vi "LOGIC_dcs.vi"(0 "image ptrs (reset - expo - subs)":u64[](array[numeric]), 1 "TotalPixels":u32, 2 "inverse":bool, 6 "write to disk":bool, 7 "Database RefNum out 2":T1, 8 "Log File":path, 9 "name":string, 11 "error in (no error)":errorcluster, 12 "reset and expo bpp":u8=16) -> (4 "image ptrs (reset - expo - subs) out":u64[](array[numeric]), 5 "bpp":i16, 10 "unsc buffer":u64, 15 "error out":errorcluster)   [LabVIEW 2016]
uses:
  DBSHAND/private/vis/DatabaseHand_RefNum.ctl
  Common/public/vis/CMN_FVAR_action.ctl
  DBSHAND/private/vis/DatabaseHand_Element_Get(bool).vi
  DBSHAND/private/vis/DatabaseHand_Element_Set(single).vi
  public/c/lib/libLogic.so
panel:
  out "output ptr (subs image)":u64
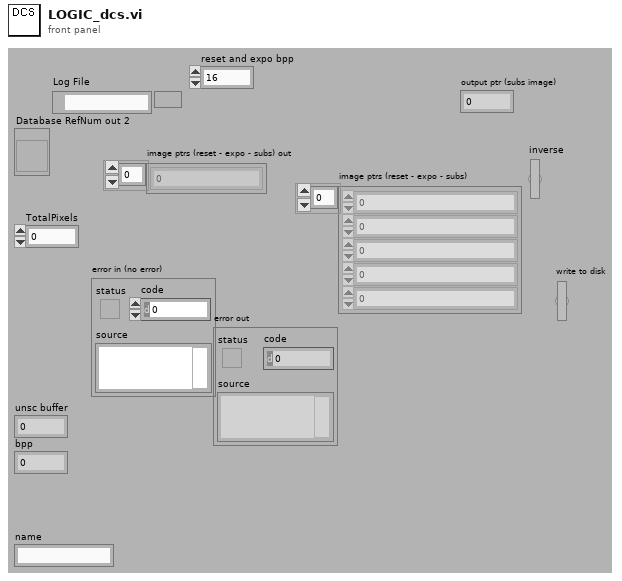
[diagram p1: front panel]
types:
  T1 = typedef "DatabaseHand_RefNum.ctl" = refnum<vi>
  T2 = typedef "CMN_FVAR_action.ctl" = enum16{"read", "write"}
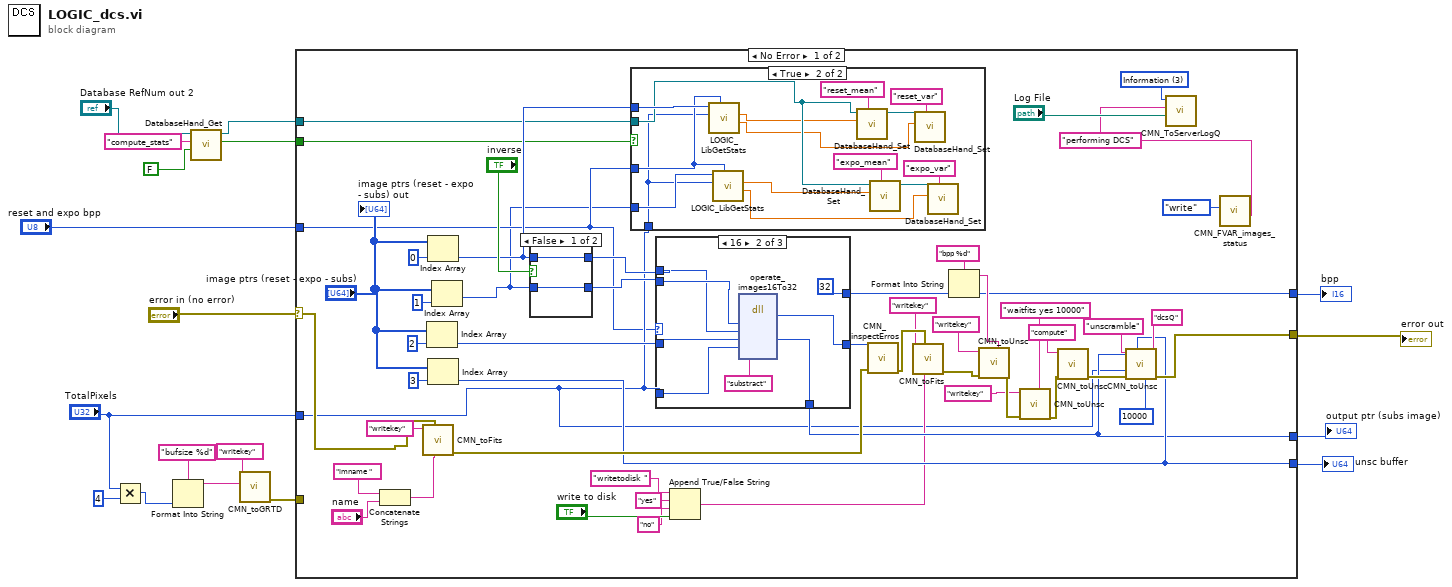
[diagram p0: block diagram]
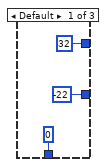
[diagram p4: hidden frame]
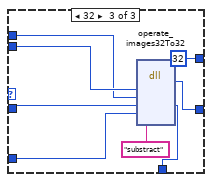
[diagram p5: hidden frame]
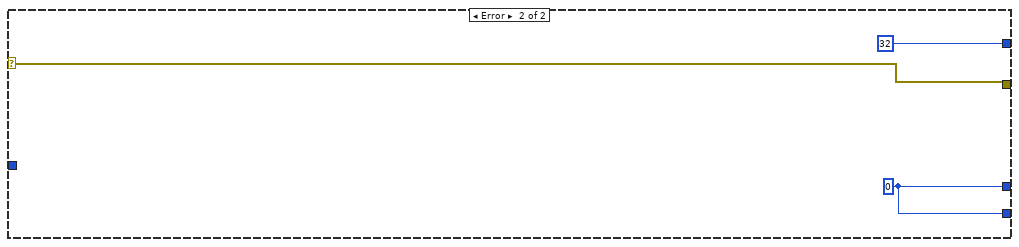
[diagram p6: hidden frame]
diagram:
  n1 = Multiply(x="TotalPixels", y=u32 4) -> (x*y=w12:u32)
  n2 = Format Into String(format string="bufsize %d", w12) -> (resulting string=w11:string)  [unwired: 2 in, 1 out]
  n3 = call-poly "DatabaseHand_Get.vi"("default value"=FALSE, "name"="compute_stats", "Database RefNum in"="Database RefNum out 2") -> ("value"=w2:bool, "Database RefNum out"=w1:T1)  [unwired: 2 in, 5 out]
  n4 = call "CMN_toGRTD.vi"("argument"=w11, "Command"="writekey") -> ("error out"=w10:errorcluster)  [unwired: 6 in, 3 out]
  n5 = case shown="No Error" "error in (no error)" {
    selector: "error in (no error)" -> [w48 w109]
    tunnel: [w65 w109] -> w7
    tunnel: "TotalPixels" -> [w23 _]
    tunnel: [w41 w108] -> w18
    tunnel: [w42 w108] -> w17
    tunnel: w10 -> [_ _]
    tunnel: [w30 32] -> w9
    tunnel: "reset and expo bpp" -> [w22 _]
    tunnel: w2 -> [w21 _]
    tunnel: w1 -> [w20 _]
    frame No Error {
      w52 = u16 3 items=["command", "imediateReply", "Callback Reply", "Information"] ("type")
      w26 = "performing DCS" ("image status")
      n6 = Concatenate Strings("imname " ("key"), "name") -> (w44:string)
      n7 = call "CMN_toFits.vi"("key"=w44, "error in (no error)"=w48, "command"="writekey") -> ("error out"=w47:errorcluster)  [unwired: 5 in, 3 out]
      n8 = Index Array(array="image ptrs (reset - expo - subs)", index=2 ("Index")) -> (element=w51:u64)
      n9 = Index Array(array="image ptrs (reset - expo - subs)", index=0 ("Index")) -> (element=w24:u64)
      n10 = Index Array(array="image ptrs (reset - expo - subs)", index=3 ("Index")) -> (element=w42:u64)
      n11 = Index Array(array="image ptrs (reset - expo - subs)", index=1 ("Index")) -> (element=w19:u64)
      n12 = case shown="False" "inverse" {
        tunnel: w24 -> [w85 w87]
        tunnel: [w85 w86] -> w28
        tunnel: w19 -> [w84 w86]
        tunnel: [w84 w87] -> w27
        frame False {
        }
        frame True {
        }
      }
      n13 = case shown="True" w21 {
        tunnel: w24 -> [_ w83]
        tunnel: w23 -> [_ w73]
        tunnel: w22 -> [_ w74]
        tunnel: w20 -> [_ w76]
        tunnel: w19 -> [_ w75]
        frame False {
        }
        frame True {
          n14 = call "LOGIC_LibGetStats.vi"("bpp"=w74, "num_elems"=w73, "imageptr"=w83) -> ("var"=w69:sgl, "mean"=w70:sgl)  [unwired: 7 out]
          n15 = call "LOGIC_LibGetStats.vi"("bpp"=w74, "num_elems"=w73, "imageptr"=w75) -> ("var"=w71:sgl, "mean"=w72:sgl)  [unwired: 7 out]
          n16 = call-poly "DatabaseHand_Set.vi"("name"="reset_mean", "value"=w70, "Database RefNum in"=w76) -> ("Database RefNum out"=w82:T1)  [unwired: 5 in, 3 out]
          n17 = call-poly "DatabaseHand_Set.vi"("name"="expo_mean", "value"=w72, "Database RefNum in"=w76) -> ("Database RefNum out"=w79:T1)  [unwired: 5 in, 3 out]
          n18 = call-poly "DatabaseHand_Set.vi"("name"="reset_var", "value"=w69, "Database RefNum in"=w82) -> ()  [unwired: 5 in, 4 out]
          n19 = call-poly "DatabaseHand_Set.vi"("name"="expo_var", "value"=w71, "Database RefNum in"=w79) -> ()  [unwired: 5 in, 4 out]
        }
      }
      n20 = case shown="16" w22 {
        tunnel: w23 -> [_ w98 w106]
        tunnel: w51 -> [_ w92 w100]
        tunnel: w28 -> [_ w93 w101]
        tunnel: w27 -> [_ w94 w102]
        tunnel: [-22 w96 w104] -> w63
        tunnel: [32 32 32] -> w30
        tunnel: [u64 0 ("imageptr3") w91 w99] -> w41
        frame Default {
        }
        frame 16 {
          n21 = dll-call lib="home/simager/panview/PAN/Modules/Logical/public/c/lib/libLogic.so" fn="operate_images16To32"("image1ptr"=w94, "image2ptr"=w93, "imageptr3"=w92, "num_elems"=w98, "operation"="substract") -> ("return type"=w96:i32, "imageptr3"=w91:u64)  [unwired: 6 in, 3 out]
        }
        frame 32 {
          n22 = dll-call lib="home/simager/panview/PAN/Modules/Logical/public/c/lib/libLogic.so" fn="operate_images32To32"("image1ptr"=w102, "image2ptr"=w101, "imageptr3"=w100, "num_elems"=w106, "operation"="substract") -> ("return type"=w104:i32, "imageptr3"=w99:u64)  [unwired: 6 in, 3 out]
        }
      }
      n23 = Append True/False String(1:"write to disk", 2:"no" ("false string"), 3:"yes" ("true string"), 4:"writetodisk " ("string (\"\")")) -> (0:w31:string)
      n24 = call "CMN_inspectErros.vi"("error in (no error)"=w47, "error code"=w63) -> ("error out"=w56:errorcluster)  [unwired: 3 in, 6 out]
      n25 = call "CMN_toFits.vi"("key"=w31, "error in (no error)"=w56, "command"="writekey") -> ("error out"=w55:errorcluster)  [unwired: 5 in, 3 out]
      n26 = Format Into String(format string="bpp %d" ("key"), w30) -> (resulting string=w49:string)  [unwired: 2 in, 1 out]
      n27 = call "CMN_toUnsc.vi"("key"=w49, "error in (no error)"=w55, "command"="writekey") -> ("error out"=w40:errorcluster)  [unwired: 6 in, 2 out]
      n28 = call "CMN_toUnsc.vi"("key"="waitfits yes 10000", "error in (no error)"=w40, "command"="writekey") -> ("error out"=w39:errorcluster)  [unwired: 6 in, 2 out]
      n29 = call "CMN_toUnsc.vi"("error in (no error)"=w39, "command"="compute") -> ("error out"=w61:errorcluster)  [unwired: 7 in, 2 out]
      n30 = call "CMN_toUnsc.vi"("responseQ"="dcsQ" ("key"), "ms timeout (-1)"=10000, "location 2"=w42, "error in (no error)"=w61, "ele Read"=w23, "location"=w41, "command"="unscramble") -> ("error out"=w65:errorcluster)  [unwired: 2 in, 2 out]
      n31 = call "CMN_ToServerLogQ.vi"("file"="Log File", "string"=w26, "type"=w52) -> ()  [unwired: 3 in, 5 out]
      n32 = call "CMN_FVAR_images_status.vi"("value in"=w26, "action"=CMN_FVAR_action."write") -> ()  [unwired: 9 out]
      "image ptrs (reset - expo - subs) out" <- "image ptrs (reset - expo - subs)"
    }
    frame Error {
      w108 = u32 0 ("Numeric")
    }
  }
  "error out" <- w7
  "output ptr (subs image)" <- w18
  "unsc buffer" <- w17
  "bpp" <- w9
